vi "zadanie_2.vi"() -> ()   [LabVIEW 2020]
panel:
  out "stan wyjscia":bool
  out "?":dynamicdata(graph)
  in  "?":bool
  in  "Amplituda":dbl(slide) scale=0.0..5.0
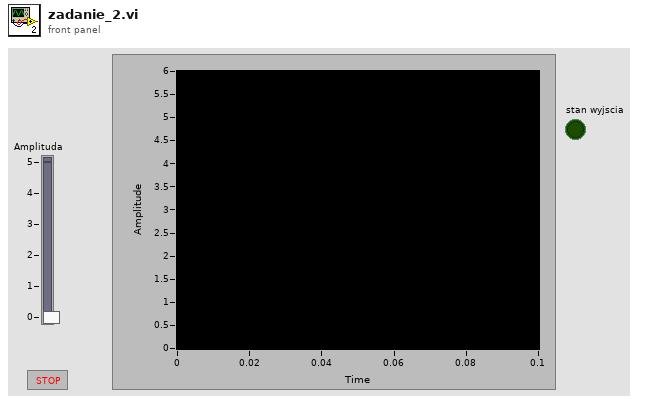
[diagram p1: front panel]
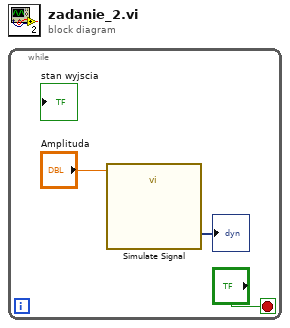
[diagram p0: block diagram]
diagram:
  n1 = while {
    stop <- "?" stop-if-true
    n2 = call "Simulate Signal"("Offset"="Amplituda") -> ("DC with Uniform Noise"=→"?":dynamicdata)  [unwired: 13 in, 1 out]
  }
